vi "ADI_IMU_ADIS16448_Open.vi"(5 "Calibrate On Open":bool=TRUE, 7 "Calibration Time (s)":dbl=3.0, 8 "error in":errorcluster, 9 "AHRS Algorithm":enum16{"Complementary", "Madgwick"}(ring), 10 "Yaw Axis":enum16{"X", "Y", "Z"}(ring)=enum."Z", 11 "SPI Chip Select":T2=enum."SPI MXP") -> (0 "error out":errorcluster, 2 "Offset Compensated Data Out":dbl[](array[numeric]), 3 "ADI IMU DevRef Out":T1={"DevStatus"={"status"=FALSE, "code"=0, "source"=""}, "Handle"=0, "SPI Bus"=enum."SPI On-Board, CS0", "Device Found"=FALSE, "Device Ready"=FALSE, "Yaw Axis"=enum."Z", "AHRS Algorithm"=enum."Complementary", "Serial"=0, "Lot ID 2"=0, "Lot ID 1"=0, "Bytes Per Sample"=0, "Calibrate On Open?"=FALSE})   [LabVIEW 2018, in "ADIS16448_IMU.lvlib"]
doc: "Initiates communication between an Analog Devices MXP IMU and the RoboRIO."
uses:
  ADIS16448_IMU.lvlib
  <vilib>/Rock Robotics/SystemInterfaces/spilib/spi_bus.ctl
  ADI_IMU_ADIS16448_IMUDevRef.ctl
  <vilib>/Rock Robotics/WPI/SPI/WPI_SPIMode.ctl
  <vilib>/Rock Robotics/SystemInterfaces/DIO/FPGA_DIOChannel.ctl
  ADI_IMU_ADIS16448_Registers.ctl
  <vilib>/Rock Robotics/SystemInterfaces/NetworkCommunication/NetComm_UsageReport_ResourceType.ctl
  <vilib>/Rock Robotics/WPI/Counter/WPI_CounterDigitalInputToDigitalSource.vi
  ADI_IMU_ADIS16448_Loop.vi
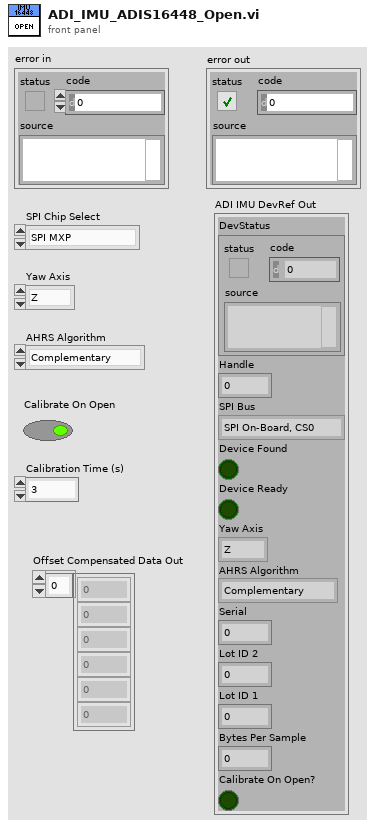
[diagram p1: front panel]
types:
  T1 = typedef "ADIS16448_IMU.lvlib/ADI_IMU_ADIS16448_IMUDevRef.ctl" = cluster{"DevStatus":errorcluster, "Handle":i32, "SPI Bus":T2, "Device Found":bool, "Device Ready":bool, "Yaw Axis":enum16{"X", "Y", "Z"}, "AHRS Algorithm":enum16{"Complementary", "Madgwick"}, "Serial":u16, "Lot ID 2":u16, "Lot ID 1":u16, "Bytes Per Sample":u16, "Calibrate On Open?":bool}
  T2 = typedef "spi_bus.ctl" = enum16{"SPI On-Board, CS0", "SPI On-Board, CS1", "SPI On-Board, CS2", "SPI On-Board, CS3", "SPI MXP", "Invalid"}
  T3 = typedef "FPGA_DIOChannel.ctl" = enum8{"DIO 0", "DIO 1", "DIO 2", "DIO 3", "DIO 4", "DIO 5", "DIO 6", "DIO 7", "DIO 8", "DIO 9", "DIO MXP 0", "DIO MXP 1", "DIO MXP 2", "DIO MXP 3", "DIO MXP 4", "DIO MXP 5", "DIO MXP 6", "DIO MXP 7", "DIO MXP 8", "DIO MXP 9", "DIO MXP 10", "DIO MXP 11", "DIO MXP 12", "DIO MXP 13", "DIO MXP 14", "DIO MXP 15", "SPI Port CS1", "SPI Port CS2", "SPI Port CS3", "SPI Port MISO", "SPI Port MOSI", "Invalid"}
  T4 = typedef "WPI_SPIMode.ctl" = enum16{"Mode 0 (Clk Idle Low,Sample on Leading)", "Mode 1 (Clk Idle Low,Sample on Trailing)", "Mode 2 (Clk Idle High,Sample on Leading)", "Mode 3 (Clk Idle High,Sample on Trailing)"}
  T5 = typedef "NetComm_UsageReport_ResourceType.ctl" = enum8{"Controller", "Module", "Language", "CANPlugin", "Accelerometer", "ADXL345", "AnalogChannel", "AnalogTrigger", "AnalogTriggerOutput", "CANJaguar", "Compressor", "Counter", "Dashboard", "DigitalInput", "DigitalOutput", "DriverStationCIO", "DriverStationEIO", "DriverStationLCD", "Encoder", "GearTooth", "Gyro", "I2C", "Framework", "Jaguar", "Joystick", "Kinect", "KinectStick", "PIDController", "Preferences", "PWM", "Relay", "RobotDrive", "SerialPort", "Servo", "Solenoid", "SPI", "Task", "Ultrasonic", "Victor", "Button", "Command", "AxisCamera", "PCVideoServer", "SmartDashboard", "Talon", "HiTechnicColorSensor", "HiTechnicAccel", "HiTechnicCompass", "SRF08", "AnalogOutput", "Victor SP", "Talon SRX", "CAN Talon SRX", "ADXL362 Accel", "ADXRS450 Gyro", "Rev SPARK", "Mindsensors SD540", "Digital Filter", "ADIS16448", "PDP", "PCM", "PigeonIMU", "Nidec Brushless", "CTRE CANifier", "CTRE Future 0", "CTRE Future 1", "CTRE Future 2", "CTRE Future 3", "CTRE Future 4", "CTRE Future 5", "CTRE Future 6", "Linear Filter", "Xbox Controller", "USB Camera", "NavX", "Pixy", "Pixy2", "ScanseSweep", "Shuffleboard", "CAN", "Digilent DMC60", "PWM Victor SPX", "Rev SPARK MAX PWM", "Rev SPARK MAX CAN", "ADIS16470"}
  T6 = typedef "ADIS16448_IMU.lvlib/ADI_IMU_ADIS16448_Registers.ctl" = u8
  T7 = typedef "WPI_DigitalOutputDevRef.ctl" = cluster{"DIO Channel":T3, "DevStatus":errorcluster}
  T8 = typedef "WPI_DigitalInputDevRef.ctl" = cluster{"DevStatus":errorcluster, "DIO Channel":T3}
  T9 = typedef "WPI_SPIDevRef.ctl" = cluster{"DevStatus":errorcluster, "Handle":i32, "SPI Bus":T2}
  T10 = typedef "FPGA_CounterEncoderSourceConvertionLVSourceType.ctl" = cluster{"DevStatus":errorcluster, "AnalogTriggerMode?":bool, "DigitalMode":cluster{"DIO Channel":T11}, "AnalogTriggerMode":cluster{"AnalogTriggerIndex":T12, "OutputType":T13}}
  T11 = typedef "FPGA_DIODigitalSourceChannel.ctl" = enum8{"DIO 0", "DIO 1", "DIO 2", "DIO 3", "DIO 4", "DIO 5", "DIO 6", "DIO 7", "DIO 8", "DIO 9", "DIO MXP 0", "DIO MXP 1", "DIO MXP 2", "DIO MXP 3", "DIO MXP 4", "DIO MXP 5", "DIO MXP 6", "DIO MXP 7", "DIO MXP 8", "DIO MXP 9", "DIO MXP 10", "DIO MXP 11", "DIO MXP 12", "DIO MXP 13", "DIO MXP 14", "DIO MXP 15", "SPI Port CS1", "SPI Port CS2", "SPI Port CS3", "SPI Port MISO", "SPI Port MOSI", "Disabled"}
  T12 = typedef "FPGA_AnalogTriggerIndex.ctl" = enum8{"Trig 0", "Trig 1", "Trig 2", "Trig 3", "Trig 4", "Trig 5", "Trig 6", "Trig 7", "Invalid"}
  T13 = typedef "FPGA_AnalogTriggerOutType.ctl" = enum16{"InWindow", "TriggerState", "Rising", "Falling"}
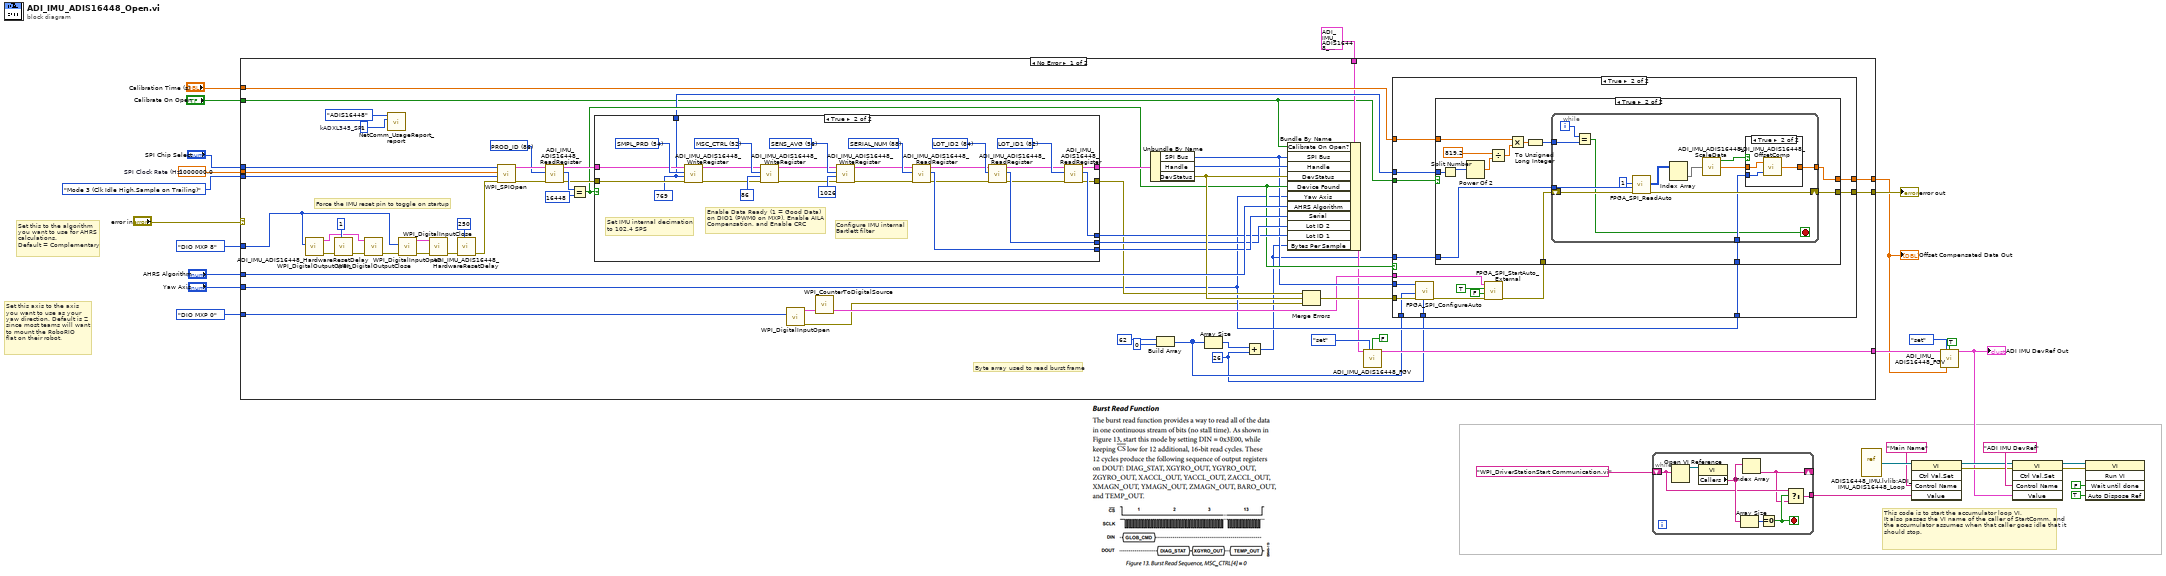
[diagram p0: block diagram]
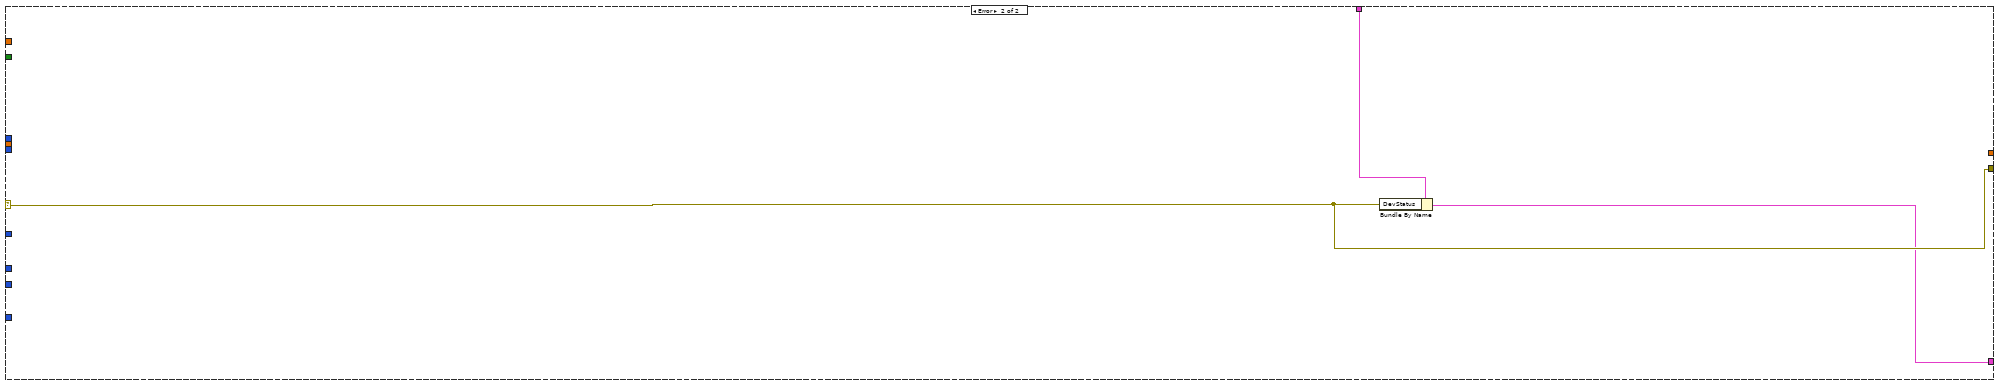
[diagram p6: hidden frame]
diagram:
  w28 = 1000000.0  # SPI Clock Rate (Hz)
  # "This code is to start the accumulator loop VI.\nIt also passes the VI name of the caller of StartComm, and the accumulator assumes when that caller goes idle that it should stop."
  # "Set this to the algorithm\nyou want to use for AHRS\ncalculations. \nDefault = Complementary"
  # "Set this axis to the axis\nyou want to use as your\nyaw direction. Default is Z\nsince most teams will want \nto mount the RoboRIO\nflat on their robot."
  n1 = case shown="No Error" "error in" {
    selector: "error in" -> [_ w161]
    tunnel: w28 -> [w83 _]
    tunnel: WPI_SPIMode."Mode 3 (Clk Idle High,Sample on Trailing)" ("Mode (3)") -> [w82 _]
    tunnel: "SPI Chip Select" -> [w81 _]
    tunnel: FPGA_DIOChannel."DIO MXP 0" ("DIO Channel") -> [w58 _]
    tunnel: "Yaw Axis" -> [w53 _]
    tunnel: "AHRS Algorithm" -> [w80 _]
    tunnel: FPGA_DIOChannel."DIO MXP 8" ("DIO Channel") -> [w79 _]
    tunnel: "Calibrate On Open" -> [w32 _]
    tunnel: "Calibration Time (s)" -> [w54 _]
    tunnel: T1 {"DevStatus"={"status"=FALSE, "code"=0, "source"=""}, "Handle"=0, "SPI Bus"=enum."SPI On-Board, CS0", "Device Found"=FALSE, "Device Ready"=FALSE, "Yaw Axis"=enum."Z", "AHRS Algorithm"=enum."Complementary", "Serial"=0, "Lot ID 2"=0, "Lot ID 1"=0, "Bytes Per Sample"=0, "Calibrate On Open?"=FALSE} ("SimpleGyroDevRef 2") -> [w52 w162]
    tunnel: [w51 w161] -> w6
    tunnel: [w47 w160] -> w3
    tunnel: [w46 _] -> w2
    frame No Error {
      w29 = 26 ("dimension size")
      w72 = u8 1  # kADXL345_SPI
      w68 = T6 86 items=["GLOB_CMD"=62, "SEQ_CNT"=58, "SMPL_PRD"=54, "SENS_AVG"=56, "MSC_CTRL"=52, "ERROR_FLAGS"=60, "TEMP"=44, "BARO"=40, "Z_MAG"=36, "Y_MAG"=32, "X_MAG"=28, "Z_ACCEL"=24, "Y_ACCEL"=20, "X_ACCEL"=16, "Z_GYRO"=12, "Y_GYRO"=8, "X_GYRO"=4, "PROD_ID"=86, "LOT_ID2"=84, "LOT_ID1"=82, "SERIAL_NUM"=88] ("ADIS16448 Register")
      # "Byte array used to read burst frame"
      # "Force the IMU reset pin to toggle on startup"
      n2 = call <vilib>:"WPI_DigitalOutputOpen.vi"("DIO Channel"=w79) -> ("error out"=w43:errorcluster, "DigitalOutputDevRef"=w37:T7)  [unwired: 9 in]
      n3 = call "ADI_IMU_ADIS16448_HardwareResetDelay.vi"("Delay (ms)"=u32 1, "error in"=w43) -> ("error out"=w44:errorcluster)  [unwired: 9 in]
      n4 = call <vilib>:"WPI_DigitalOutputClose.vi"("error in (no error)"=w44, "DigitalOutputDevRef"=w37) -> ("error out"=w42:errorcluster)  [unwired: 9 in]
      n5 = call <vilib>:"NetComm_UsageReport_report.vi"("Instance Number"=w72, "Resource Type"=NetComm_UsageReport_ResourceType."ADIS16448") -> ()  [unwired: 10 in]
      n6 = call <vilib>:"WPI_DigitalInputOpen.vi"("error in (no error)"=w42, "DIO Channel"=w79) -> ("error out"=w41:errorcluster, "DigitalInputDevRef"=w40:T8)  [unwired: 8 in]
      n7 = call <vilib>:"WPI_DigitalInputClose.vi"("error in (no error)"=w41, "DigitalInputDevRef"=w40) -> ("error out"=w39:errorcluster)  [unwired: 9 in]
      n8 = call "ADI_IMU_ADIS16448_HardwareResetDelay.vi"("Delay (ms)"=u32 250, "error in"=w39) -> ("error out"=w73:errorcluster)  [unwired: 9 in]
      n9 = call <vilib>:"WPI_SPIOpen.vi"("error in"=w73, "Mode (3)"=w82, "Clock Rate (Hz)"=w83, "SPI Bus"=w81) -> ("error out"=w69:errorcluster, "SPIDevRef"=w70:T9)  [unwired: 6 in]
      n10 = call "ADI_IMU_ADIS16448_ReadRegister.vi"("error in (no error)"=w69, "ADIS16448 Register"=w68, "SPIDevRef in"=w70) -> ("error out"=w64:errorcluster, "Register Value"=w67:u16, "SPIDevRef out"=w65:T9)  [unwired: 6 in]
      n11 = Equal?(x=w67, y=u16 16448) -> (x = y?=w60:bool)
      n12 = case shown="True" w60 {
        tunnel: [_ w153] -> w76
        tunnel: [_ w152] -> w75
        tunnel: [_ w150] -> w74
        tunnel: [w133 w138] -> w63
        tunnel: [w132 w137] -> w62
        tunnel: w65 -> [w133 w136]
        tunnel: w64 -> [w132 w135]
        tunnel: [_ w134] -> w55
        frame False {
        }
        frame True {
          w149 = T6 82 items=["GLOB_CMD"=62, "SEQ_CNT"=58, "SMPL_PRD"=54, "SENS_AVG"=56, "MSC_CTRL"=52, "ERROR_FLAGS"=60, "TEMP"=44, "BARO"=40, "Z_MAG"=36, "Y_MAG"=32, "X_MAG"=28, "Z_ACCEL"=24, "Y_ACCEL"=20, "X_ACCEL"=16, "Z_GYRO"=12, "Y_GYRO"=8, "X_GYRO"=4, "PROD_ID"=86, "LOT_ID2"=84, "LOT_ID1"=82, "SERIAL_NUM"=88] ("ADIS16448 Register")
          w151 = T6 84 items=["GLOB_CMD"=62, "SEQ_CNT"=58, "SMPL_PRD"=54, "SENS_AVG"=56, "MSC_CTRL"=52, "ERROR_FLAGS"=60, "TEMP"=44, "BARO"=40, "Z_MAG"=36, "Y_MAG"=32, "X_MAG"=28, "Z_ACCEL"=24, "Y_ACCEL"=20, "X_ACCEL"=16, "Z_GYRO"=12, "Y_GYRO"=8, "X_GYRO"=4, "PROD_ID"=86, "LOT_ID2"=84, "LOT_ID1"=82, "SERIAL_NUM"=88] ("ADIS16448 Register")
          w154 = T6 88 items=["GLOB_CMD"=62, "SEQ_CNT"=58, "SMPL_PRD"=54, "SENS_AVG"=56, "MSC_CTRL"=52, "ERROR_FLAGS"=60, "TEMP"=44, "BARO"=40, "Z_MAG"=36, "Y_MAG"=32, "X_MAG"=28, "Z_ACCEL"=24, "Y_ACCEL"=20, "X_ACCEL"=16, "Z_GYRO"=12, "Y_GYRO"=8, "X_GYRO"=4, "PROD_ID"=86, "LOT_ID2"=84, "LOT_ID1"=82, "SERIAL_NUM"=88] ("ADIS16448 Register")
          w155 = T6 56 items=["GLOB_CMD"=62, "SEQ_CNT"=58, "SMPL_PRD"=54, "SENS_AVG"=56, "MSC_CTRL"=52, "ERROR_FLAGS"=60, "TEMP"=44, "BARO"=40, "Z_MAG"=36, "Y_MAG"=32, "X_MAG"=28, "Z_ACCEL"=24, "Y_ACCEL"=20, "X_ACCEL"=16, "Z_GYRO"=12, "Y_GYRO"=8, "X_GYRO"=4, "PROD_ID"=86, "LOT_ID2"=84, "LOT_ID1"=82, "SERIAL_NUM"=88] ("ADIS16448 Register")
          w156 = T6 52 items=["GLOB_CMD"=62, "SEQ_CNT"=58, "SMPL_PRD"=54, "SENS_AVG"=56, "MSC_CTRL"=52, "ERROR_FLAGS"=60, "TEMP"=44, "BARO"=40, "Z_MAG"=36, "Y_MAG"=32, "X_MAG"=28, "Z_ACCEL"=24, "Y_ACCEL"=20, "X_ACCEL"=16, "Z_GYRO"=12, "Y_GYRO"=8, "X_GYRO"=4, "PROD_ID"=86, "LOT_ID2"=84, "LOT_ID1"=82, "SERIAL_NUM"=88] ("ADIS16448 Register")
          w157 = T6 54 items=["GLOB_CMD"=62, "SEQ_CNT"=58, "SMPL_PRD"=54, "SENS_AVG"=56, "MSC_CTRL"=52, "ERROR_FLAGS"=60, "TEMP"=44, "BARO"=40, "Z_MAG"=36, "Y_MAG"=32, "X_MAG"=28, "Z_ACCEL"=24, "Y_ACCEL"=20, "X_ACCEL"=16, "Z_GYRO"=12, "Y_GYRO"=8, "X_GYRO"=4, "PROD_ID"=86, "LOT_ID2"=84, "LOT_ID1"=82, "SERIAL_NUM"=88] ("ADIS16448 Register")
          w134 = u16 769 ("Data")
          # "Configure IMU internal\nBartlett filter"
          # "Enable Data Ready (1 = Good Data) \non DIO1 (PWM0 on MXP), Enable AILA\nCompensation, and Enable CRC"
          # "Set IMU internal decimation\nto 102.4 SPS"
          n13 = call "ADI_IMU_ADIS16448_WriteRegister.vi"("error in (no error)"=w135, "Data"=w134, "ADIS16448 Register"=w157, "SPIDevRef in"=w136) -> ("error out"=w147:errorcluster, "SPIDevRef out"=w148:T9)  [unwired: 6 in]
          n14 = call "ADI_IMU_ADIS16448_WriteRegister.vi"("error in (no error)"=w147, "Data"=u16 86, "ADIS16448 Register"=w156, "SPIDevRef in"=w148) -> ("error out"=w145:errorcluster, "SPIDevRef out"=w146:T9)  [unwired: 6 in]
          n15 = call "ADI_IMU_ADIS16448_WriteRegister.vi"("error in (no error)"=w145, "Data"=u16 1026, "ADIS16448 Register"=w155, "SPIDevRef in"=w146) -> ("error out"=w143:errorcluster, "SPIDevRef out"=w144:T9)  [unwired: 6 in]
          n16 = call "ADI_IMU_ADIS16448_ReadRegister.vi"("error in (no error)"=w143, "ADIS16448 Register"=w154, "SPIDevRef in"=w144) -> ("error out"=w141:errorcluster, "Register Value"=w153:u16, "SPIDevRef out"=w142:T9)  [unwired: 6 in]
          n17 = call "ADI_IMU_ADIS16448_ReadRegister.vi"("error in (no error)"=w141, "ADIS16448 Register"=w151, "SPIDevRef in"=w142) -> ("error out"=w139:errorcluster, "Register Value"=w152:u16, "SPIDevRef out"=w140:T9)  [unwired: 6 in]
          n18 = call "ADI_IMU_ADIS16448_ReadRegister.vi"("error in (no error)"=w139, "ADIS16448 Register"=w149, "SPIDevRef in"=w140) -> ("error out"=w137:errorcluster, "Register Value"=w150:u16, "SPIDevRef out"=w138:T9)  [unwired: 6 in]
        }
      }
      n19 = call <vilib>:"WPI_DigitalInputOpen.vi"("DIO Channel"=w58) -> ("error out"=w36:errorcluster, "DigitalInputDevRef"=w57:T8)  [unwired: 9 in]
      n20 = call-poly <vilib>:"WPI_CounterToDigitalSource.vi"("DigitalInputDevRef"=w57) -> ("Digital Source"=w56:T10)  [unwired: 6 in]
      n21 = Unbundle By Name(w63) -> ("SPI Bus"=w59:T2, "Handle"=w78:i32, "DevStatus"=w77:errorcluster)
      n22 = Build Array(u8 62 ("hi"), u8 0 ("element")) -> (w33:u8[])
      n23 = Array Size(array=w33) -> (size(s)=w31:i32)
      n24 = Add(x=w31, y=w29) -> (x+y=w30:i32)
      n25 = Bundle By Name(cluster=w52, "Calibrate On Open?"=w32, "SPI Bus"=w59, "Handle"=w78, "DevStatus"=w77, "Device Found"=w60, "Yaw Axis"=w53, "AHRS Algorithm"=w80, "Serial"=w76, "Lot ID 2"=w75, "Lot ID 1"=w74, "Bytes Per Sample"=w30) -> (w48:T1)
      n26 = Merge Errors(w62, w77, w36) -> (w61:errorcluster)
      n27 = call "ADI_IMU_ADIS16448_FGV.vi"("ADI IMU DevRef"=w48, "Operation"=enum16{"set", "get", "set reset"}."set", "Sensor Ready?"=FALSE) -> ("ADI IMU DevRef Out"=w47:T1)  [unwired: 6 in, 6 out]
      n28 = case shown="True" w60 {
        tunnel: w61 -> [w84 w100]
        tunnel: w59 -> [_ w99]
        tunnel: w33 -> [_ w87]
        tunnel: w56 -> [_ w95]
        tunnel: w32 -> [_ w94]
        tunnel: w55 -> [_ w92]
        tunnel: w54 -> [_ w91]
        tunnel: [_ w90] -> w46
        tunnel: w53 -> [_ w89]
        tunnel: [w84 w88] -> w51
        tunnel: w30 -> [_ w86]
        tunnel: w29 -> [_ w85]
        frame False {
        }
        frame True {
          n29 = call <vilib>:"FPGA_SPI_ConfigureAuto.vi"("SPI Auto Zero Byte Count"=w85, "error in"=w100, "SPI Auto TX Byte Array"=w87, "SPI Bus"=w99) -> ("error out"=w98:errorcluster)  [unwired: 7 in]
          n30 = call <vilib>:"FPGA_SPI_StartAuto_External.vi"("error in (no error)"=w98, "Falling Edge"=FALSE, "Rising Edge"=TRUE, "Source"=w95) -> ("error out"=w93:errorcluster)  [unwired: 7 in]
          n31 = case shown="True" w94 {
            tunnel: w93 -> [w101 w114]
            tunnel: w92 -> [_ w113]
            tunnel: w91 -> [_ w108]
            tunnel: [_ w106] -> w90
            tunnel: w89 -> [_ w107]
            tunnel: [w101 w105] -> w88
            tunnel: w86 -> [_ w102]
            frame False {
            }
            frame True {
              n32 = Split Number(x=w113) -> (hi(x)=w104:u8)  [unwired: 1 out]
              n33 = Power Of 2(x=w104) -> (2^x=w111:dbl)
              n34 = Divide(x=819.2, y=w111) -> (x/y=w110:dbl)
              n35 = Multiply(x=w108, y=w110) -> (x*y=w109:dbl)
              n36 = To Unsigned Long Integer(number=w109) -> (unsigned 32bit integer=w103:u32)
              n37 = while {
                shift-right: [w126] -> w105
                shift-left: w114 -> [w127]
                tunnel: w107 -> [w125]
                tunnel: [w124] -> w106
                tunnel: w102 -> [w122]
                tunnel: w103 -> [w119]
                i -> [w120]
                stop <- w118 stop-if-true
                n38 = Equal?(x=w120, y=w119) -> (x = y?=w118:bool)
                n39 = call <vilib>:"FPGA_SPI_ReadAuto.vi"("error in (no error)"=w127, "Bytes per Sample"=w122, "Samples to Read"=u32 1) -> ("error out"=w126:errorcluster, "Data"=w117:u8[][])  [unwired: 6 in, 1 out]
                n40 = Index Array(array=w117) -> (element=w116:u8[])  [unwired: 2 in]
                n41 = call "ADI_IMU_ADIS16448_ScaleData.vi"("Received Data"=w116) -> ("Data Array"=w123:dbl[], "Data Good?"=w115:bool)  [unwired: 3 in]
                n42 = case shown="True" w115 {
                  tunnel: w125 -> [_ w131]
                  tunnel: [w128 w130] -> w124
                  tunnel: w123 -> [w128 w129]
                  frame False {
                  }
                  frame True {
                    n43 = call "ADI_IMU_ADIS16448_OffsetComp.vi"("Yaw Axis"=w131, "Raw Data"=w129) -> ("Offset Compensated Data"=w130:dbl[])
                  }
                }
              }
            }
          }
        }
      }
    }
    frame Error {
      n44 = Bundle By Name(cluster=w162, "DevStatus"=w161) -> (w160:T1)
    }
  }
  "error out" <- w6
  "Offset Compensated Data Out" <- w2
  n45 = while {
    shift-right: [w164] -> _
    shift-left: "WPI_DriverStationStart Communication.vi" -> [w165]
    tunnel: [w163] -> w12
    stop <- w166 stop-if-true
    n46 = Open VI Reference(vi path=w165) -> (vi reference=w169:refnum<vi>)  [unwired: 1 in, 5 out]
    n47 = property class="VI"(reference=w169) -> ("Callers"=w167:string[])  [unwired: 1 in, 2 out]
    n48 = Array Size(array=w167) -> (size(s)=w168:i32)
    n49 = Index Array(array=w167) -> (element=w164:string)  [unwired: 1 in]
    n50 = Equal To 0?(x=w168) -> (x = 0?=w166:bool)
    n51 = Select(t=w165, s=w166, f=w164) -> (s? t:f=w163:string)
  }
  n52 = vi-ref "ADIS16448_IMU.lvlib:ADI_IMU_ADIS16448_Loop.vi"() -> (w14:refnum<vi>)
  n53 = invoke class="VI" method="Ctrl Val.Set"(reference=w14, "Control Name"="Main Name", "Value"=w12) -> (reference out=w11:refnum<vi>, error out=w16:errorcluster)  [unwired: 2 in, 3 out]
  n54 = call "ADI_IMU_ADIS16448_FGV.vi"("ADI IMU DevRef"=w3, "Operation"=enum16{"set", "get", "set reset"}."set", "Sensor Ready?"=TRUE, "Offset Compensated Data"=w2) -> ("ADI IMU DevRef Out"=w1:T1)  [unwired: 5 in, 6 out]
  "ADI IMU DevRef Out" <- w1
  n55 = invoke class="VI" method="Ctrl Val.Set"(reference=w11, error in=w16, "Control Name"="ADI IMU DevRef", "Value"=w1) -> (reference out=w21:refnum<vi>, error out=w17:errorcluster)  [unwired: 1 in, 3 out]
  n56 = invoke class="VI" method="Run VI"(reference=w21, error in=w17, "Wait until done"=FALSE ("Wait Until Done"), "Auto Dispose Ref"=TRUE ("Auto Dispose Reference")) -> ()  [unwired: 1 in, 5 out]
